vi "mirrorTestInterface.vi"() -> ()   [LabVIEW 2016]
uses:
  <vilib>/Platform/TimedLoop/XDataNode/timing_clust.ctl
  <vilib>/Platform/TimedLoop/XDataNode/nitl_modes.ctl
  <vilib>/Platform/TimedLoop/XDataNode/wakeup.ctl
  <vilib>/platform/TimedLoop/XDataNode/XDataNode.xnode
  <vilib>/Platform/TimedLoop/XDataNode/XDNodeRunTimeDep.lvlib
panel:
  out "length":i32
  in  "y":dbl
  in  "x":dbl
  in  "stop":bool
  out "bytes written":i32
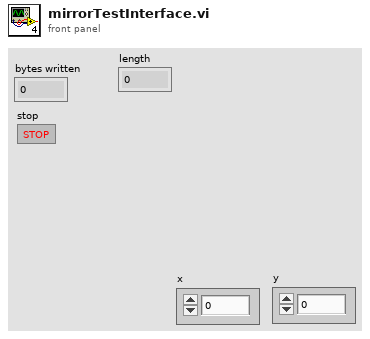
[diagram p1: front panel]
types:
  T1 = typedef "XDNodeRunTimeDep.lvlib/timing_clust.ctl" = cluster{"Expected End [f-1]":u64, "Actual End [f-1]":u64, "Finished Late? [f-1]":bool, "Expected End [i-1]":u64, "Actual End [i-1]":u64, "Finished Late? [i-1]":bool, "Expected Start [i]":u64, "Actual Start [i]":u64, "Expected Start [f]":u64, "Actual Start [f]":u64, "Source Name":string, "Structure Name":string, "Period":i64, "Deadline":i64, "Offset":i64, "Start":i64, "Priority":i32, "Timeout":i32, "Mode":T2, "Wakeup Reason":T3, "Error":errorcluster, "Source Type":string, "Secondary Source Type":string, "Global End Time":u64, "Global Start Time":u64, "Frame Duration":u64, "Iteration Duration":u64, "Assigned CPU":i32, "I/O Scan Engine Mode":u32}
  T2 = typedef "XDNodeRunTimeDep.lvlib/nitl_modes.ctl" = enum32{"No Change", "Process missed periods, maintain original phase", "Discard missed periods, maintain original phase", "Process missed periods, ignore original phase", "Discard missed periods, ignore original phase"}
  T3 = typedef "XDNodeRunTimeDep.lvlib/wakeup.ctl" = enum32{"Normal", "Aborted", "Asynchronous wakeup", "Timing source error", "Timed loop error", "Timeout"}
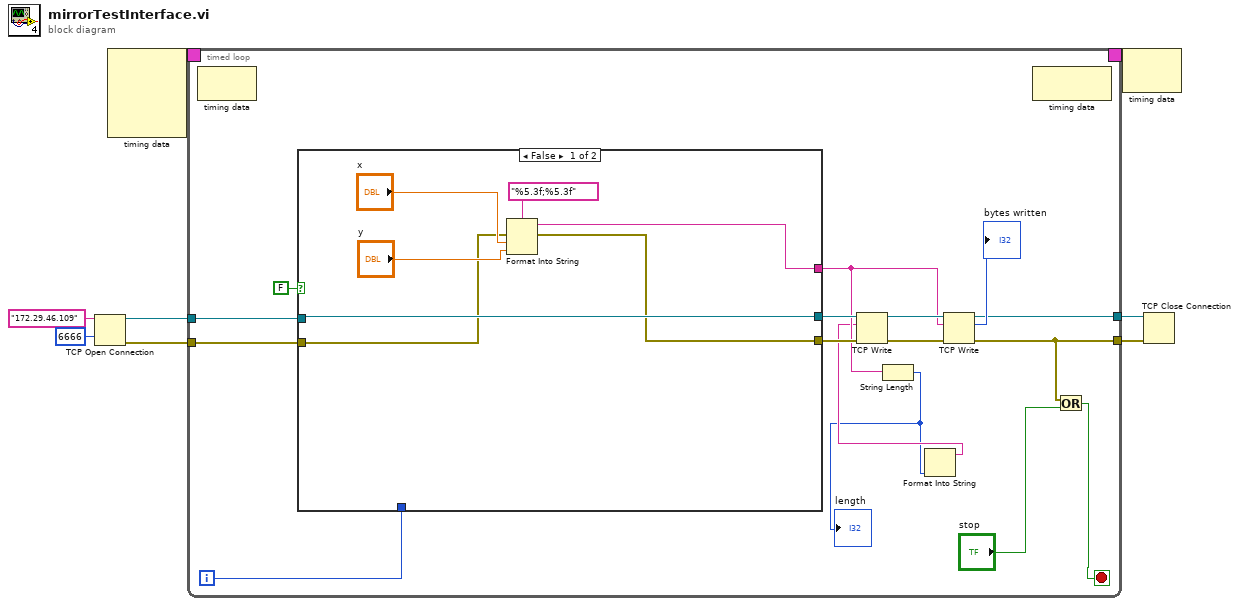
[diagram p0: block diagram]
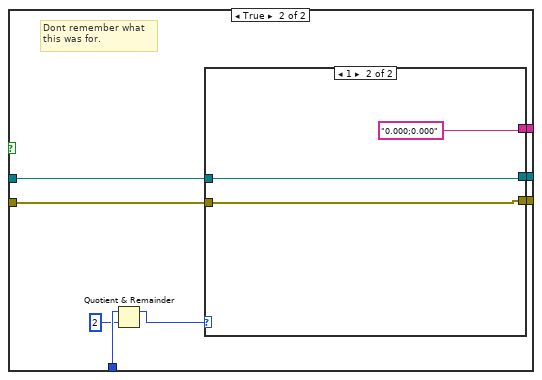
[diagram p2: hidden frame]
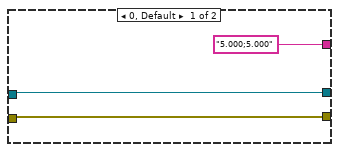
[diagram p3: hidden frame]
diagram:
  n1 = TCP Open Connection(address="172.29.46.109", remote port or service name=u16 6666) -> (connection ID=w4:refnum<k5>, error out=w3:errorcluster)  [unwired: 3 in]
  n2 = node-c288() -> (w8:T1)  [unwired: 4 in]
  n3 = timed-loop {
    timing: w8 -> [_]
    timing-out: [_] -> w7
    tunnel: w4 -> [w23]
    tunnel: w3 -> [w22]
    tunnel: [w16] -> w1
    tunnel: [w15] -> w2
    i -> [w24]
    stop <- w14 stop-if-true
    n4 = node-c288() -> ()  [unwired: 1 in, 1 out]
    n5 = case shown="False" FALSE {
      tunnel: w24 -> [_ w39]
      tunnel: w23 -> [w31 w37]
      tunnel: w22 -> [w27 w36]
      tunnel: [w31 w35] -> w21
      tunnel: [w25 w34] -> w20
      tunnel: [w26 w33] -> w11
      frame False {
        n6 = Format Into String(format string="%5.3f;%5.3f", error in=w27, "x", "y") -> (resulting string=w26:string, error out=w25:errorcluster)  [unwired: 1 in]
      }
      frame True {
        # "Dont remember what\nthis was for."
        n7 = Quotient & Remainder(x=w39, y=2) -> (x-y*floor(x/y)=w32:i32)  [unwired: 1 out]
        n8 = case shown="1" w32 {
          tunnel: w37 -> [w42 w44]
          tunnel: w36 -> [w41 w43]
          tunnel: [w42 w44] -> w35
          tunnel: [w41 w43] -> w34
          tunnel: ["5.000;5.000" "0.000;0.000"] -> w33
          frame 0, Default {
          }
          frame 1 {
          }
        }
      }
    }
    n9 = String Length(string=w11) -> (length=w9:i32)
    "length" <- w9
    n10 = Format Into String(w9) -> (resulting string=w10:string)  [unwired: 3 in, 1 out]
    n11 = TCP Write(connection ID=w21, data in=w10, error in (no error)=w20) -> (connection ID out=w18:refnum<k5>, error out=w19:errorcluster)  [unwired: 1 in, 1 out]
    n12 = TCP Write(connection ID=w18, data in=w11, error in (no error)=w19) -> (connection ID out=w16:refnum<k5>, bytes written=→"bytes written":i32, error out=w15:errorcluster)  [unwired: 1 in]
    n13 = node-c288() -> ()  [unwired: 1 in, 1 out]
    n14 = Or(x=w15, y="stop") -> (x .or. y?=w14:bool)
  }
  n15 = node-c288(w7) -> ()  [unwired: 1 out]
  n16 = TCP Close Connection(connection ID=w1, error in (no error)=w2) -> ()  [unwired: 1 in, 2 out]
